vi "2photocell+ledcontrol+sum_cal3.vi"() -> ()   [LabVIEW 2016]
uses:
  <vilib>/LabVIEW Interface for Arduino/LabVIEW Interface for Arduino.lvlib
  <vilib>/ptbypt/NI_PtbyPt.lvlib
panel:
  in  "stop":bool
  in  "Tab Control":enum32{"Page 1", "Page 2", "Page 3"}(tab)
  out "Voltage 1":dbl(knob) scale=0.0..5.0
  out "Filtered x 2":dbl format="%0.2f"
  out "alarm":bool
  out "LUX":string="Error"
  out "Voltage 2":dbl(knob) scale=0.0..5.0
  out "Filtered x 1":dbl format="%0.2f"
  in  "br_coef":dbl
  in  "thrs low":i32=1
  in  "thrs high":i32=4
  in  "q":dbl
  in  "p":dbl
  in  "k":dbl
  in  "thrs up":dbl
  in  "thrs down":dbl
  in  "Slide 3":dbl(slide) min=0.0 max=255.0 scale=0.0..255.0
  in  "Slide 2":dbl(slide) min=0.0 max=255.0 scale=0.0..255.0
  in  "Slide":dbl(slide) min=0.0 max=255.0 scale=0.0..255.0
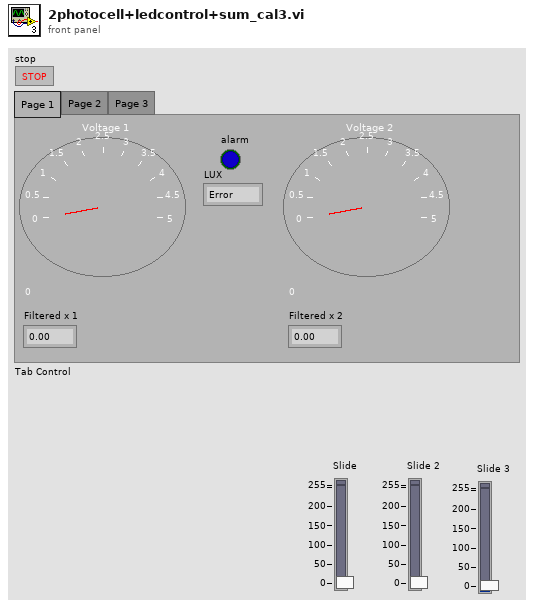
[diagram p1: front panel]
types:
  T1 = typedef "LabVIEW Interface for Arduino.lvlib/Arduino Resource.ctl" = cluster{"VISA resource":refnum<visa-resource-name>, "Board Type":T2, "Connection Type":enum8{"USB / Serial"}, "Bytes Per Packet (15)":u8}
  T2 = typedef "LabVIEW Interface for Arduino.lvlib/Board Type.ctl" = enum16{"Uno", "Dimuelanove w/Atmega 328", "Mega 2560"}
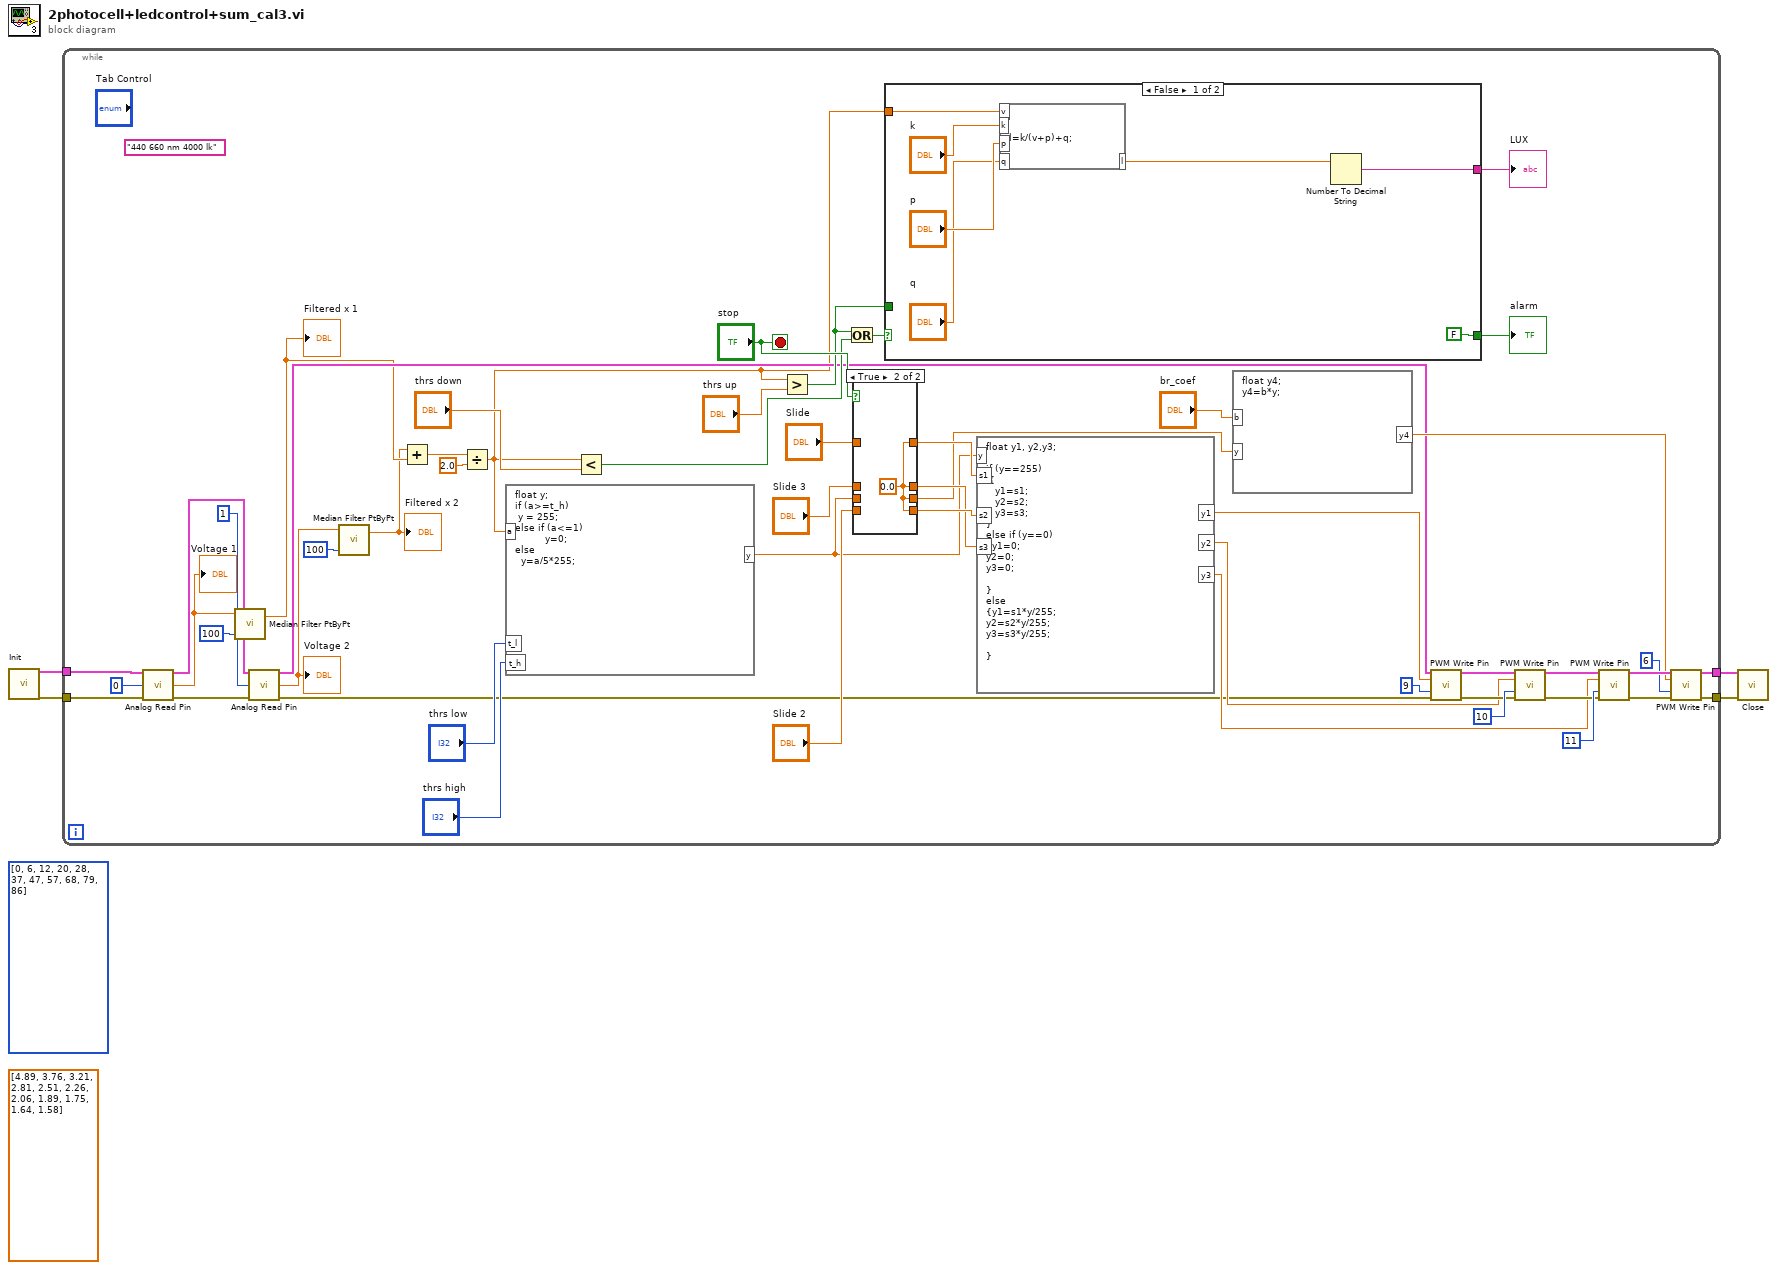
[diagram p0: block diagram]
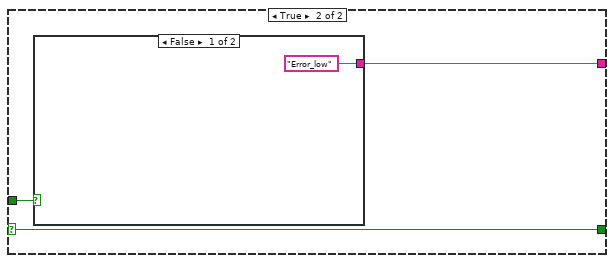
[diagram p2: hidden frame]
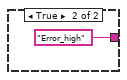
[diagram p3: hidden frame]
diagram:
  (unwired) dbl[] [4.89, 3.76, 3.21, 2.81, 2.51, 2.26, 2.06, 1.89, 1.75, 1.64, 1.58]
  (unwired) i32[] [0, 6, 12, 20, 28, 37, 47, 57, 68, 79, 86]
  n1 = call <vilib>:"Init.vi"() -> ("Arduino Resource"=w3:T1, "error out"=w4:errorcluster)  [unwired: 18 in]
  n2 = while {
    tunnel: w4 -> [w55]
    tunnel: w3 -> [w17]
    tunnel: [w32] -> w2
    tunnel: [w31] -> w1
    stop <- "stop" stop-if-true
    (unwired) "440 660 nm 4000 lk"
    n3 = call <vilib>:"Analog Read Pin.vi"("Arduino Resource"=w17, "Analog Input Pin (0)"=u8 0, "error in"=w55) -> ("Arduino Resource"=w16:T1, "Voltage"=w53:dbl, "error out"=w14:errorcluster)  [unwired: 10 in]
    "Voltage 1" <- w53
    n4 = call <vilib>:"Median Filter PtByPt.vi"("rank"=100, "x"=w53) -> ("Filtered x"=w6:dbl)  [unwired: 2 in, 1 out]
    "Filtered x 1" <- w6
    n5 = call <vilib>:"Analog Read Pin.vi"("Arduino Resource"=w16, "Analog Input Pin (0)"=u8 1, "error in"=w14) -> ("Arduino Resource"=w15:T1, "Voltage"=w10:dbl, "error out"=w13:errorcluster)  [unwired: 10 in]
    "Voltage 2" <- w10
    n6 = call <vilib>:"Median Filter PtByPt.vi"("rank"=100, "x"=w10) -> ("Filtered x"=w5:dbl)  [unwired: 2 in, 1 out]
    "Filtered x 2" <- w5
    n7 = Add(x=w5, y=w6) -> (x+y=w8:dbl)
    n8 = Divide(x=w8, y=2.0) -> (x/y=w7:dbl)
    n9 = formula code="float y;\nif (a>=t_h)\n y = 255;\nelse if (a<=1)\n          y=0;\nelse\n  y=a/5*255;"("a"=w7, "t_l"="thrs low", "t_h"="thrs high") -> ("y"=w28:dbl)
    n10 = Less?(x=w7, y="thrs down") -> (x < y?=w22:bool)
    n11 = Greater?(x=w7, y="thrs up") -> (0:w18:bool)
    n12 = Or(x=w18, y=w22) -> (x .or. y?=w21:bool)
    n13 = case shown="True" "stop" {
      tunnel: "Slide 2" -> [w72 _]
      tunnel: [w72 w73] -> w38
      tunnel: "Slide 3" -> [w71 _]
      tunnel: [w71 w73] -> w37
      tunnel: "Slide" -> [w70 _]
      tunnel: [w70 w73] -> w39
      tunnel: w28 -> [w69 _]
      tunnel: [w69 w73] -> w26
      frame False {
      }
      frame True {
        w73 = 0.0 ("Slide 2")
      }
    }
    n14 = case shown="False" w21 {
      selector: w21 -> [_ w66]
      tunnel: [FALSE w66] -> w20
      tunnel: w7 -> [w62 _]
      tunnel: [w60 w64] -> w19
      tunnel: w18 -> [_ w65]
      frame False {
        n15 = formula code="l=k/(v+p)+q;"("v"=w62, "k"="k", "p"="p", "q"="q") -> ("l"=w61:dbl)
        n16 = Number To Decimal String(number=w61) -> (decimal integer string=w60:string)  [unwired: 1 in]
      }
      frame True {
        n17 = case shown="False" w65 {
          tunnel: ["Error_low" "Error_high"] -> w64
          frame False {
          }
          frame True {
          }
        }
      }
    }
    "alarm" <- w20
    "LUX" <- w19
    n18 = formula code="float y1, y2,y3;\n\nif (y==255)\n {\n   y1=s1;\n   y2=s2;\n   y3=s3;\n}\nelse if (y==0)\n{y1=0;\ny2=0;\ny3=0;\n\n}\nelse \n{y1=s1*y/255;\ny2=s2*y/255;\ny3=s3*y/255;\n\n}"("s1"=w39, "s2"=w38, "s3"=w37, "y"=w28) -> ("y1"=w36:dbl, "y2"=w35:dbl, "y3"=w34:dbl)
    n19 = formula code="float y4;\ny4=b*y;"("b"="br_coef", "y"=w26) -> ("y4"=w25:dbl)
    n20 = call <vilib>:"PWM Write Pin.vi"("Arduino Resource"=w15, "Duty Cycle (0 - 255)"=w36, "PWM Pin (3)"=u8 9, "error in"=w13) -> ("Arduino Resource"=w45:T1, "error out"=w41:errorcluster)  [unwired: 10 in]
    n21 = call <vilib>:"PWM Write Pin.vi"("Arduino Resource"=w45, "Duty Cycle (0 - 255)"=w35, "PWM Pin (3)"=u8 10, "error in"=w41) -> ("Arduino Resource"=w44:T1, "error out"=w40:errorcluster)  [unwired: 10 in]
    n22 = call <vilib>:"PWM Write Pin.vi"("Arduino Resource"=w44, "Duty Cycle (0 - 255)"=w34, "PWM Pin (3)"=u8 11, "error in"=w40) -> ("Arduino Resource"=w33:T1, "error out"=w30:errorcluster)  [unwired: 10 in]
    n23 = call <vilib>:"PWM Write Pin.vi"("Arduino Resource"=w33, "Duty Cycle (0 - 255)"=w25, "PWM Pin (3)"=u8 6, "error in"=w30) -> ("Arduino Resource"=w32:T1, "error out"=w31:errorcluster)  [unwired: 10 in]
  }
  n24 = call <vilib>:"Close.vi"("Arduino Resource"=w2, "error in"=w1) -> ()  [unwired: 13 in, 1 out]
